vi "X-axis Range Read.vi"(4 "error in (no error)":errorcluster, 6 "Container State":T2, 7 "Display State In":T1={"Numeric"=0.0, "Fill Plots"=FALSE, "Cursor Redraw"=TRUE, "XYGraph Refnum"=refnum}) -> (0 "error out":errorcluster, 2 "Value":cluster{"Low Value":dbl, "High Value":dbl}, 3 "Display State Out":T1={"Numeric"=0.0, "Fill Plots"=FALSE, "Cursor Redraw"=TRUE, "XYGraph Refnum"=refnum})   [LabVIEW 2020, in "Overview XControl.xctl"]
uses:
  Overview XControl.xctl
  <vilib>/_xctls/Container State.ctl
  Overview State.ctl
  <vilib>/_xctls/XControlSupport.lvlib
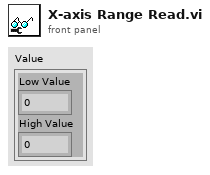
[diagram p1: front panel]
types:
  T1 = typedef "Overview XControl.xctl/Overview State.ctl" = cluster{"Numeric":dbl, "Fill Plots":bool, "Cursor Redraw":bool, "XYGraph Refnum":refnum<vi>}
  T2 = typedef "XControlSupport.lvlib/Container State.ctl" = cluster{"Indicator?":bool, "Run Mode?":bool, " Refnum":refnum<vi>}
  T3 = cluster{"XScale.Minimum":dbl, "XScale.Maximum":dbl}
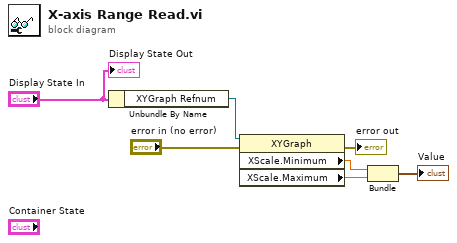
[diagram p0: block diagram]
diagram:
  n1 = Unbundle By Name("Display State In") -> ("XYGraph Refnum"=w7:refnum<vi>)
  n2 = property class="XYGraph"(reference=w7, error in="error in (no error)") -> (error out=→"error out":errorcluster, "XScale.Minimum"=w5:dbl, "XScale.Maximum"=w4:dbl)  [unwired: 1 out]
  n3 = Bundle("XScale.Minimum"=w5, "XScale.Maximum"=w4) -> (→"Value":T3)  [unwired: 1 in]
  "Display State Out" <- "Display State In"
